vi "HappyDecorator_Init.vi"(8 "error in (no error)":errorcluster, 10 "Object":refnum<class "Object.lvclass">, 11 "Object in":refnum<class "HappyDecorator.lvclass">) -> (0 "error out":errorcluster, 3 "object out":refnum<class "HappyDecorator.lvclass">)   [LabVIEW 2020, in "HappyDecorator.lvclass"]
uses:
  HappyDecorator.lvclass
  C:/Projects/DesignPatterns/DecoratorPattern2/ObjectDecorator_class/ObjectDecorator.lvclass
  Object_interface/Object.lvclass
  HappyDecorator.lvclass/HappyDecorator.ctl
  ObjectDecorator_class/ObjectDecorator.lvclass
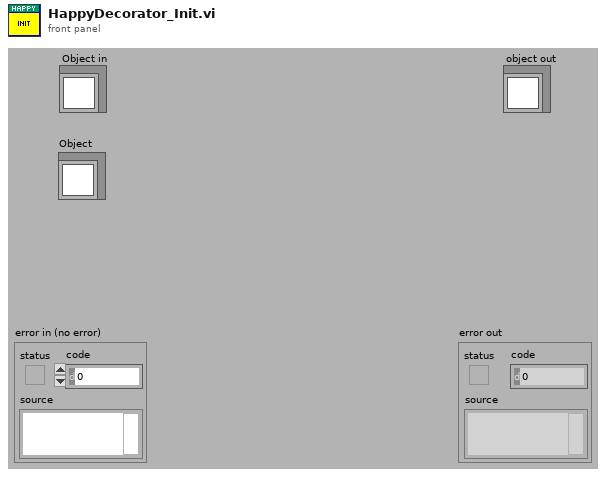
[diagram p1: front panel]
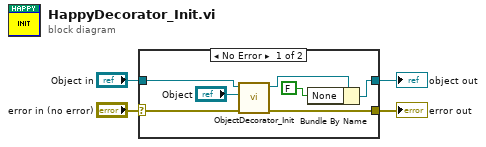
[diagram p0: block diagram]
diagram:
  n1 = case shown="No Error" "error in (no error)" {
    selector: "error in (no error)" -> [w9 w12]
    tunnel: [w11 w13] -> w4
    tunnel: "Object in" -> [w7 w13]
    tunnel: [w8 w12] -> w1
    frame No Error {
      n2 = call "ObjectDecorator_Init.vi"("error in (no error)"=w9, "Object"="Object", "object in"=w7) -> ("error out"=w8:errorcluster, "object out"=w6:refnum<class "HappyDecorator.lvclass">)  [unwired: 7 in]
      n3 = Bundle By Name(cluster=w6, "None"=FALSE) -> (w11:refnum<class "HappyDecorator.lvclass">)
    }
    frame Error {
    }
  }
  "object out" <- w4
  "error out" <- w1
